vi "dfd_Min-Max Phase Spectral Factorization (Cepstrum).vi"(8 "error in (no error)":errorcluster, 11 "numerator":dbl[](array[numeric])) -> (0 "error out":errorcluster, 1 "maximum phase":dbl[](array[numeric]), 2 "minimum phase":dbl[](array[numeric]))   [LabVIEW 2017, in "NI_DigFilter_Design.lvlib"]
doc: "Performs Min-Max phase spectral factorization by use of cepstrum of the filter."
uses:
  <vilib>/addons/Digital Filter Design/NI_DigFilter_Design.lvlib
  <vilib>/Analysis/2dsp.llb/Real FFT.vi
  <vilib>/addons/Digital Filter Design/_Misc.llb/dfd_Error Cluster From Error Code (Scalar).vi
  <vilib>/addons/Digital Filter Design/_Misc.llb/dfd_Error Handlers (Single).vi
  <vilib>/Analysis/2dsp.llb/Zero Padder (DBL).vi
  <vilib>/addons/Digital Filter Design/NI_DigFilterLicensed.lvlib
  <vilib>/Analysis/NI_AALPro.lvlib
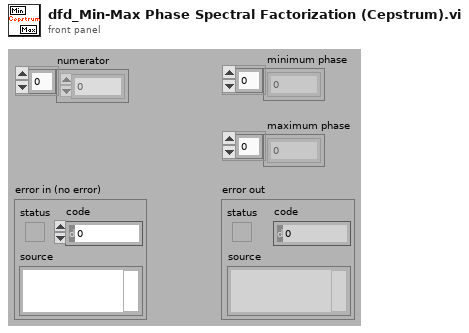
[diagram p1: front panel]
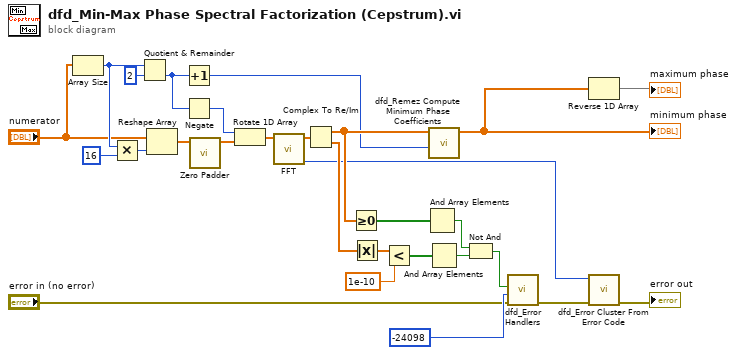
[diagram p0: block diagram]
diagram:
  n1 = Array Size(array="numerator") -> (size(s)=w27:i32)
  n2 = Multiply(x=w27, y=16) -> (x*y=w23:i32)
  n3 = Quotient & Remainder(x=w27, y=2) -> (floor(x/y)=w21:i32)  [unwired: 1 out]
  n4 = Reshape Array("numerator", w23) -> (w22:dbl[])
  n5 = Increment(x=w21) -> (x+1=w4:i32)
  n6 = Negate(x=w21) -> (-x=w18:i32)
  n7 = call-poly <vilib>:"Zero Padder.vi"("Input Array"=w22) -> ("Zero Padded Array"=w17:dbl[])  [unwired: 1 in, 9 out]
  n8 = Rotate 1D Array(1:w17, 2:w18) -> (0:w19:dbl[])
  n9 = call-poly <vilib>:"FFT.vi"("X"=w19) -> ("error"=w1:i32, "FFT {X}"=w20:cdb[])  [unwired: 2 in, 7 out]
  n10 = Complex To Re/Im(x + iy=w20) -> (x=w5:dbl[], y=w16:dbl[])
  n11 = Greater Or Equal To 0?(x=w5) -> (x >= 0?=w14:bool[])
  n12 = Absolute Value(x=w16) -> (abs(x)=w15:dbl[])
  n13 = Less?(x=w15, y=1e-10) -> (x < y?=w13:bool[])
  n14 = And Array Elements(Boolean array=w14) -> (logical AND=w12:bool)
  n15 = call <vilib>:"dfd_Remez Compute Minimum Phase Coefficients.vi"("# of taps"=w4, "H(w)"=w5) -> ("h"=w3:dbl[])  [unwired: 9 out]
  "minimum phase" <- w3
  n16 = And Array Elements(Boolean array=w13) -> (logical AND=w11:bool)
  n17 = Not And(1:w11, 2:w12) -> (0:w10:bool)
  n18 = call-poly <vilib>:"dfd_Error Handlers.vi"("error in (no error)"="error in (no error)", "error code"=-24098 ("ERR_SPECTRAL_FACTORIZATION_FAIL"), "condition failed?"=w10) -> ("error out"=w7:errorcluster)  [unwired: 8 out]
  n19 = Reverse 1D Array(array=w3) -> (reversed array=→"maximum phase":dbl[])
  n20 = call-poly <vilib>:"dfd_Error Cluster From Error Code.vi"("error in (no error)"=w7, "error code (0)"=w1) -> ("error out"=→"error out":errorcluster)  [unwired: 9 out]
